vi "超标浓度报警配置.vi"() -> ()   [LabVIEW 2016]
uses:
  <vilib>/Utility/config.llb/NI_LVConfig.lvlib
panel:
  in  "CODCr超标浓度":dbl
  in  "CODMn超标浓度":dbl
  in  "总氮超标浓度":dbl
  in  "总磷超标浓度":dbl
  in  "氨氮超标浓度":dbl
  in  "取消":bool
  in  "确认":bool
  # "超标浓度报警配置"
  # "mg/L"
  # "mg/L"
  # "mg/L"
  # "mg/L"
  # "mg/L"
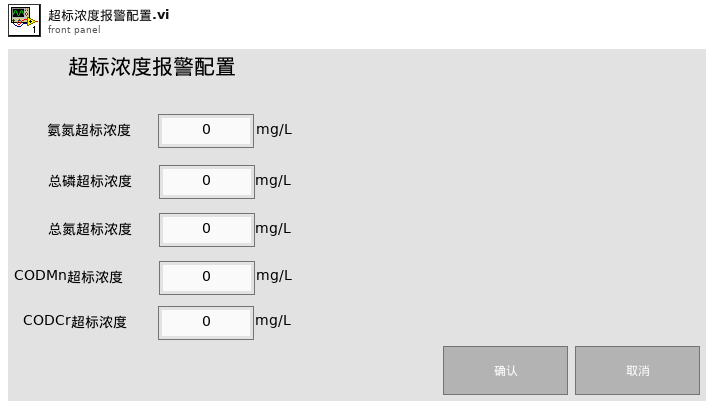
[diagram p1: front panel]
types:
  T1 = typedef "NI_LVConfig.lvlib/Config Data RefNum.ctl" = refnum<k1>
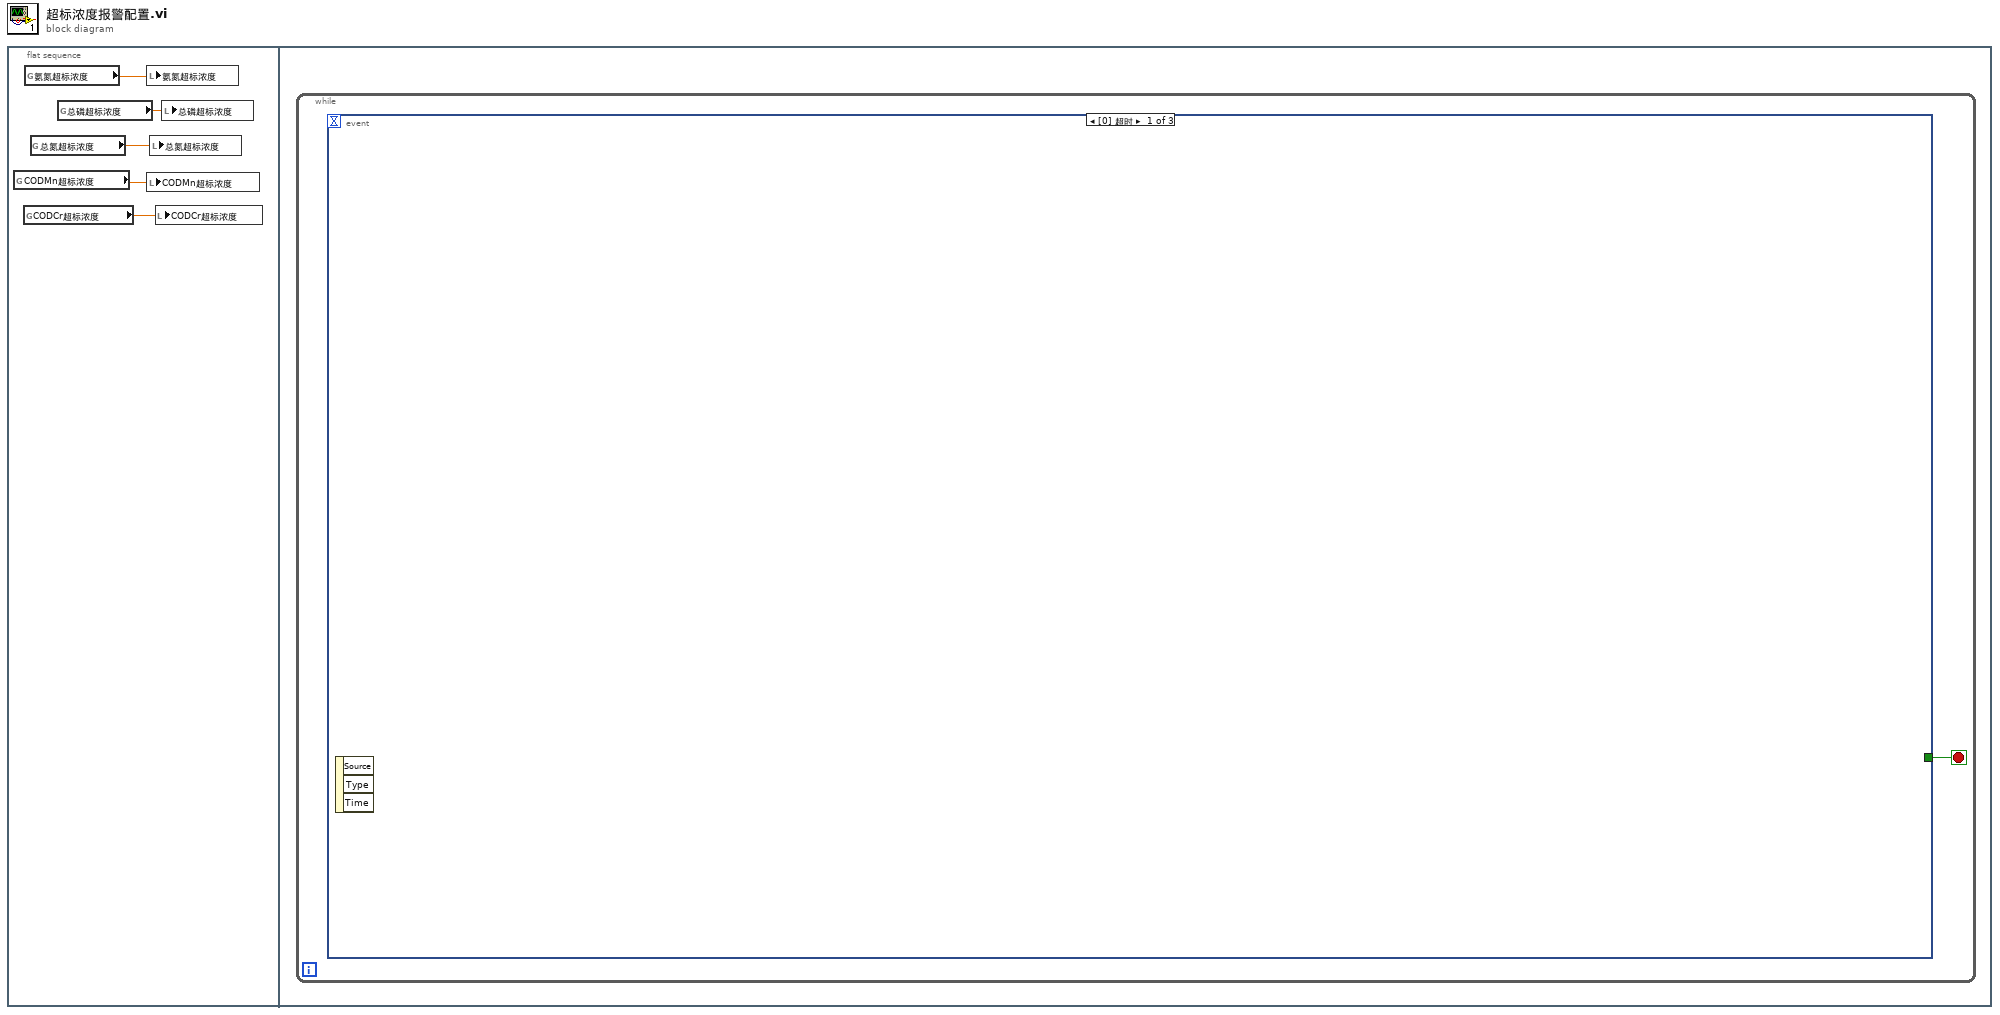
[diagram p0: block diagram]
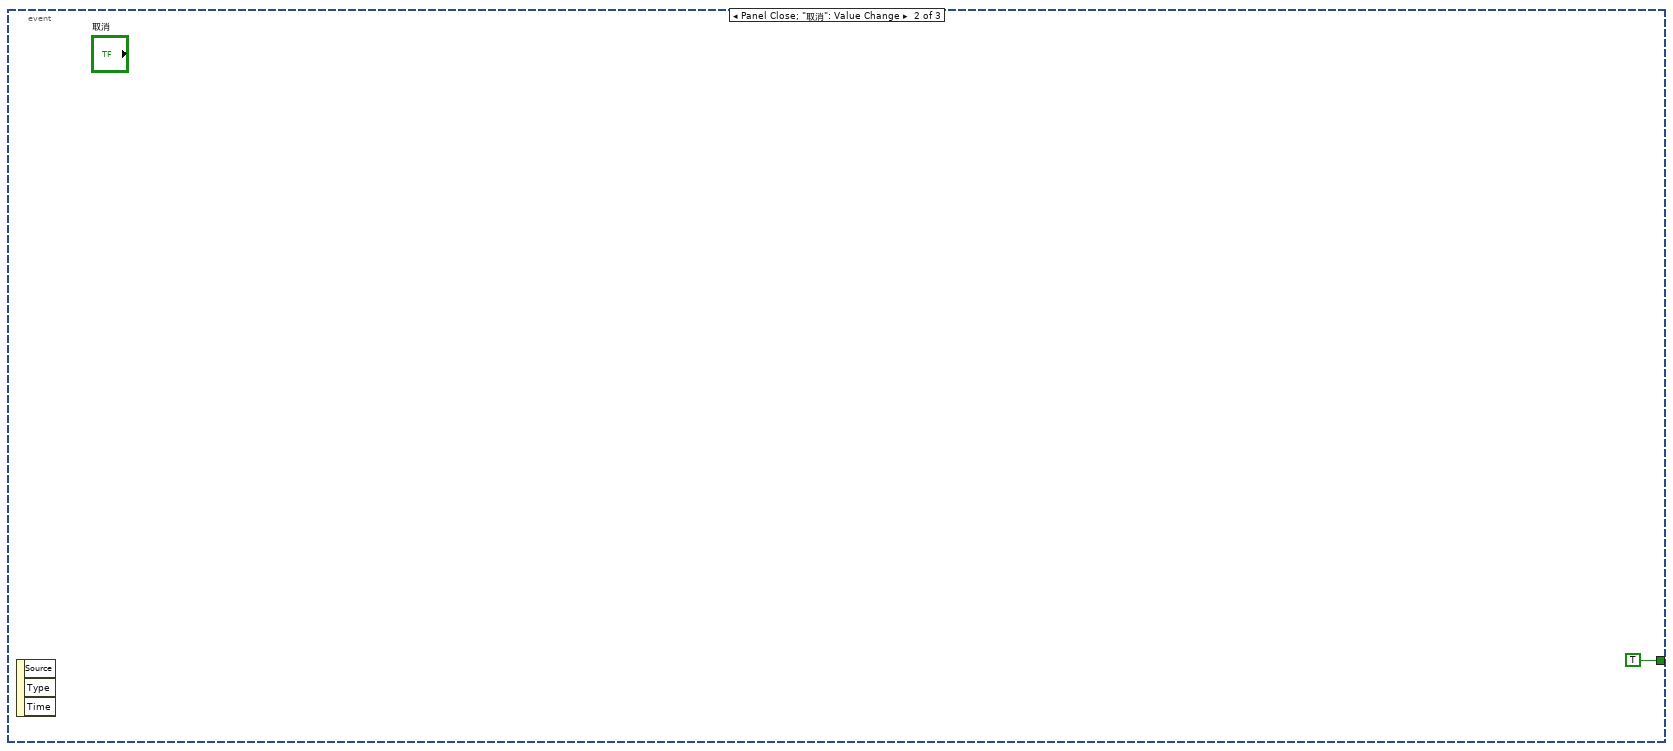
[diagram p2: hidden frame]
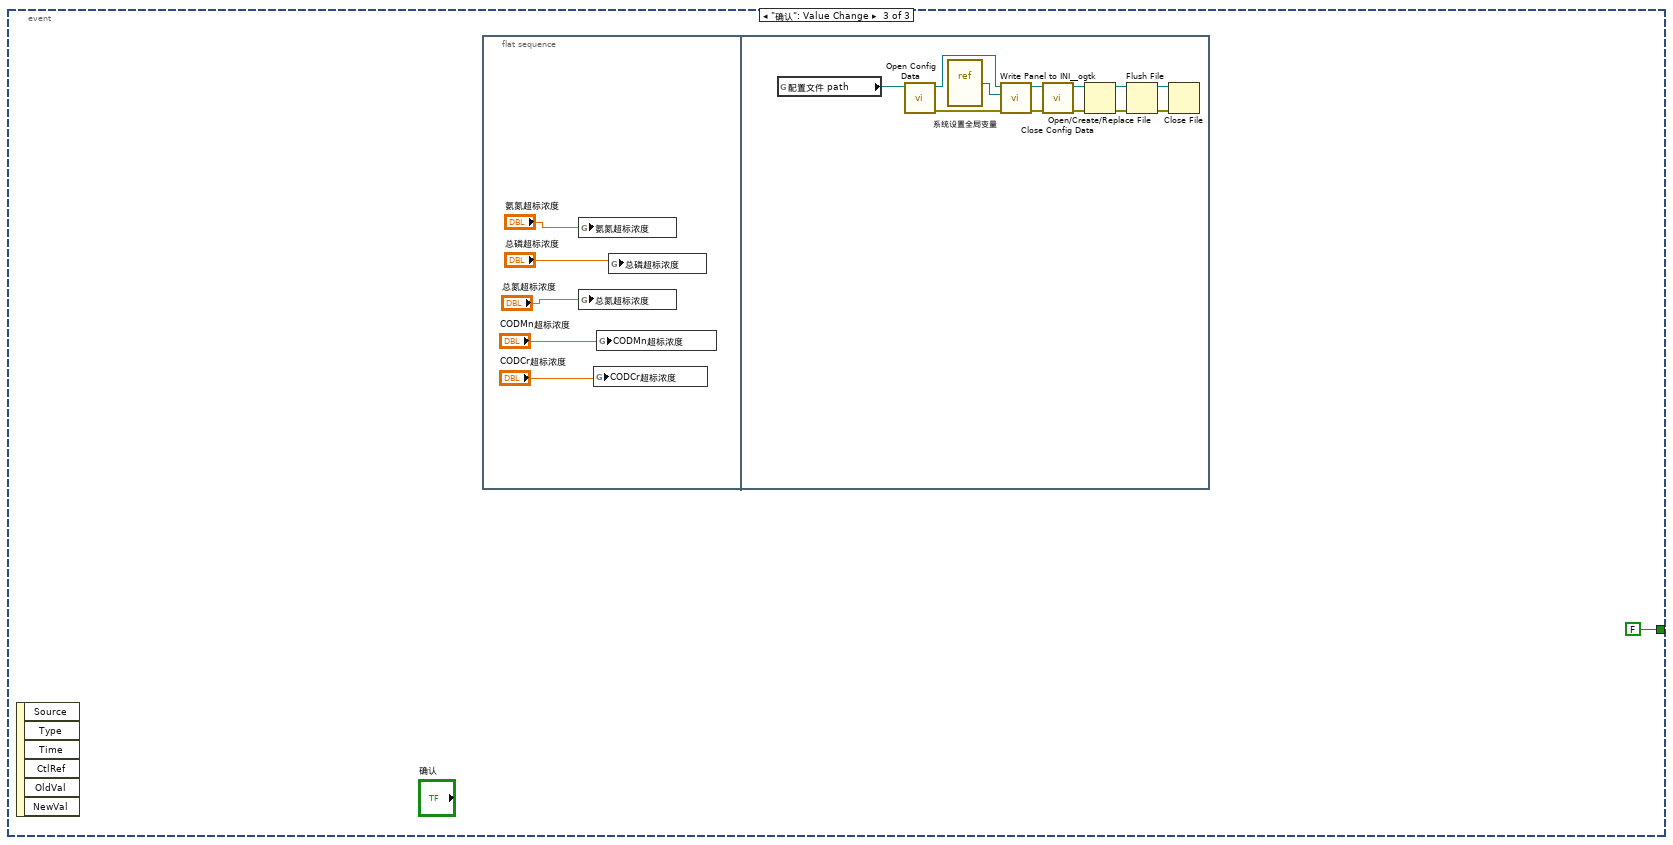
[diagram p3: hidden frame]
diagram:
  n1 = flat-sequence {
    frame #0 {
      n2 = global read "系统设置全局变量.vi" "CODMn超标浓度"() -> (w5:dbl)
      n3 = global read "系统设置全局变量.vi" "CODCr超标浓度"() -> (w2:dbl)
      n4 = global read "系统设置全局变量.vi" "氨氮超标浓度"() -> (w4:dbl)
      n5 = global read "系统设置全局变量.vi" "总氮超标浓度"() -> (w1:dbl)
      n6 = global read "系统设置全局变量.vi" "总磷超标浓度"() -> (w3:dbl)
      n7 = local write "氨氮超标浓度"(w4) -> ()
      n8 = local write "CODMn超标浓度"(w5) -> ()
      n9 = local write "总氮超标浓度"(w1) -> ()
      n10 = local write "CODCr超标浓度"(w2) -> ()
      n11 = local write "总磷超标浓度"(w3) -> ()
    }
    frame #1 {
      n12 = while {
        stop <- w6 stop-if-true
        n13 = event shown="[0] 超时" {
          selector: _ -> [_ _ _]
          dyn-events: _ -> [_ _ _]
          timeout: _ -> [_ _ _]
          tunnel: [_ TRUE FALSE] -> w6
          event Timeout {
            n14 = event-data() -> ()  [unwired: 1 in, 3 out]
          }
          event Panel Close; "取消": Value Change {
            n15 = event-data() -> ()  [unwired: 1 in, 3 out]
          }
          event "确认": Value Change {
            n16 = event-data() -> ()  [unwired: 1 in, 6 out]
            n17 = flat-sequence {
              frame #0 {
                n18 = global write "系统设置全局变量.vi" "氨氮超标浓度"("氨氮超标浓度") -> ()
                n19 = global write "系统设置全局变量.vi" "总氮超标浓度"("总氮超标浓度") -> ()
                n20 = global write "系统设置全局变量.vi" "CODCr超标浓度"("CODCr超标浓度") -> ()
                n21 = global write "系统设置全局变量.vi" "CODMn超标浓度"("CODMn超标浓度") -> ()
                n22 = global write "系统设置全局变量.vi" "总磷超标浓度"("总磷超标浓度") -> ()
              }
              frame #1 {
                n23 = global read "ping全局.vi" "配置文件 path"() -> (w14:path)
                n24 = call <vilib>:"Open Config Data.vi"("configuration file path"=w14) -> ("error out"=w22:errorcluster, "refnum"=w25:T1)  [unwired: 8 in, 1 out]
                n25 = vi-ref "系统设置全局变量.vi"() -> (w24:refnum<vi>)
                n26 = call <userlib>:"Write Panel to INI__ogtk.vi"("error in (no error)"=w22, "VI ref"=w24, "refnum"=w25) -> ("error out"=w21:errorcluster, "refnum out"=w23:T1)  [unwired: 7 in]
                n27 = call <vilib>:"Close Config Data.vi"("error in (no error)"=w21, "refnum"=w23) -> ("error out"=w16:errorcluster, "file path"=w15:path)  [unwired: 8 in]
                n28 = Open/Create/Replace File(file path (use dialog)=w15, error in=w16) -> (refnum out=w19:refnum<file>, error out=w20:errorcluster)  [unwired: 4 in, 1 out]
                n29 = Flush File(refnum=w19, error in=w20) -> (refnum out=w18:refnum<file>, error out=w17:errorcluster)
                n30 = Close File(refnum=w18, error in=w17) -> ()  [unwired: 2 out]
              }
            }
          }
        }
      }
    }
  }
